vi "Connect To Execution Engine.vi"(0 "message":string, 11 "error in":errorcluster) -> (15 "error out":errorcluster)   [LabVIEW 2023, in "RFFixtureCharact.Public.lvlib"]
uses:
  RFFixtureCharact.Public.lvlib
  Common/RFCalAndFixtureCharact.Common.lvlib
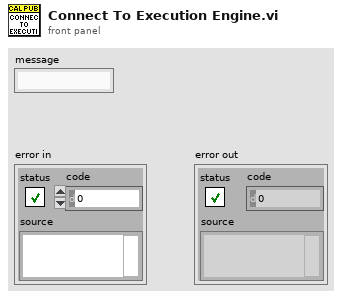
[diagram p1: front panel]
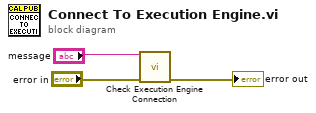
[diagram p0: block diagram]
diagram:
  n1 = call "Check Execution Engine Connection.vi"("message"="message", "error in (no error)"="error in") -> ("error out"=→"error out":errorcluster)  [unwired: 13 in]
